vi "ConvertPostionsToString.vi"(11 "positions":string[](array[string])) -> (3 "output string":string)   [LabVIEW 2014]
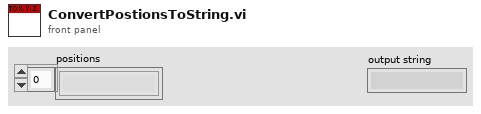
[diagram p1: front panel]
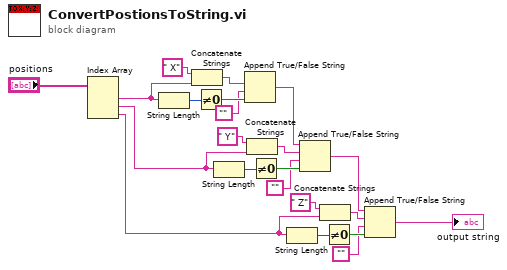
[diagram p0: block diagram]
diagram:
  n1 = Index Array(array="positions") -> (element #1=w20:string, element #2=w19:string, element #3=w18:string)  [unwired: 3 in]
  n2 = String Length(string=w20) -> (length=w13:i32)
  n3 = Concatenate Strings(" X", w20) -> (w15:string)
  n4 = Not Equal To 0?(x=w13) -> (x != 0?=w14:bool)
  n5 = String Length(string=w19) -> (length=w9:i32)
  n6 = Append True/False String(1:w14, 2:"", 3:w15) -> (0:w17:string)  [unwired: 1 in]
  n7 = Concatenate Strings(" Y", w19) -> (w11:string)
  n8 = Not Equal To 0?(x=w9) -> (x != 0?=w10:bool)
  n9 = String Length(string=w18) -> (length=w5:i32)
  n10 = Append True/False String(1:w10, 2:"", 3:w11, 4:w17) -> (0:w21:string)
  n11 = Concatenate Strings(" Z", w18) -> (w7:string)
  n12 = Not Equal To 0?(x=w5) -> (x != 0?=w6:bool)
  n13 = Append True/False String(1:w6, 2:"", 3:w7, 4:w21) -> (0:→"output string":string)
